vi "Logic.vi"(8 "error in (no error)":errorcluster, 11 "CIFTemplatePlugin in":refnum<class "CIFTemplatePlugin.lvclass">) -> (0 "error out":errorcluster, 3 "CIFTemplatePlugin out":refnum<class "CIFTemplatePlugin.lvclass">)   [LabVIEW 2021, in "CIFTemplatePlugin.lvclass"]
uses:
  CIFTemplatePlugin.lvclass
  D:/dev/CIF-LVCore/src/CIFCore/Class/CIFCorePlugin.lvclass
  CIFTemplatePlugin.lvclass/CIFTemplatePlugin.ctl
  Common/Typedef/Channels.ctl
  CIFCore/Class/CIFCorePlugin.lvclass/CIFCorePlugin.ctl
  Channels/CIFChannelMng/CIFChannelMng.lvclass/CIFChannelMng.ctl
  Channels/CIFChannels/CIFChannels.lvclass/CIFChannels.ctl
  Channels/CIFTag/Double/CIFTagDouble.lvclass/CIFTagDouble.ctl
  Channels/CIFTag/CIFTag/CIFTag.lvclass/CIFTag.ctl
  Channels/CIFTag/U64/CIFTagU64.lvclass/CIFTagU64.ctl
  CIFCore/Class/Accessors/Monitor/Write Double 1.vi
  CIFCore/Class/Accessors/Monitor/Write U64 1.vi
  CIFCore/Class/Accessors/Monitor/Write I64 1.vi
  CIFCore/Class/Accessors/Monitor/Write I64 2.vi
  Channels/CIFTag/CIFTag/Accessors/Read CIF Channel.vi
  Channels/CIFTag/CIFTag/SubVIs/Check Disconnect.vi
  Channels/CIFTag/Double/Core/Read Double_no_dd.vi/cbead010-ab61-49ec-ac6c-083511305d37.vi
  Channels/CIFTag/CIFTag/Accessors/Write CIF Channel.vi
  Channels/CIFChannels/Accessors/Read Channel State.vi
  Channels/CIFChannels/Accessors/Read Direction.vi
  Channels/CIFChannels/Accessors/Read Forced.vi
  Channels/CIFTag/U64/Core/Read U64_no_dd.vi/cbead010-ab61-49ec-ac6c-083511305d37.vi
  Channels/CIFTag/Double/Core/Write Double_no_dd.vi/e6e5dc56-0fe0-434b-816e-55c2e61471c2.vi
  Channels/CIFTag/U64/Core/Write U64_no_dd.vi/e6e5dc56-0fe0-434b-816e-55c2e61471c2.vi
  Channels/CIFChannels/Accessors/Write Channel State.vi
  Channels/CIFChannels/Accessors/Read Disconnect Behavior.vi
  Channels/CIFTag/Double/Core/Read Double_no_dd.vi/cbead010-ab61-49ec-ac6c-083511305d37.vi/c28b0ead-42ad-4072-80a2-aca7f2bd7ce3.vi
  Channels/CIFTag/Double/Core/Read Double_no_dd.vi/cbead010-ab61-49ec-ac6c-083511305d37.vi/219d0231-d98b-4193-b5cc-84f90e3c9091.vi
  <vilib>/CIFChannels/SubVIs/Get dll Path.vi
  Channels/CIFTag/U64/Core/Read U64_no_dd.vi/cbead010-ab61-49ec-ac6c-083511305d37.vi/c28b0ead-42ad-4072-80a2-aca7f2bd7ce3.vi
  Channels/CIFTag/U64/Core/Read U64_no_dd.vi/cbead010-ab61-49ec-ac6c-083511305d37.vi/219d0231-d98b-4193-b5cc-84f90e3c9091.vi
  Channels/CIFTag/Double/Core/Write Double_no_dd.vi/e6e5dc56-0fe0-434b-816e-55c2e61471c2.vi/4bc1c15b-36ab-481f-b8dd-c64075ce723a.vi
  Channels/CIFTag/Double/Core/Write Double_no_dd.vi/e6e5dc56-0fe0-434b-816e-55c2e61471c2.vi/d83cb72b-7713-41fc-a3d1-682de79cf574.vi
  Channels/CIFTag/U64/Core/Write U64_no_dd.vi/e6e5dc56-0fe0-434b-816e-55c2e61471c2.vi/4bc1c15b-36ab-481f-b8dd-c64075ce723a.vi
  Channels/CIFTag/U64/Core/Write U64_no_dd.vi/e6e5dc56-0fe0-434b-816e-55c2e61471c2.vi/d83cb72b-7713-41fc-a3d1-682de79cf574.vi
  Channels/CIFTag/CIFTag/CIFTag.lvclass
  D:/dev/CIF-LVCore/src/Channels/CIFChannels/CIFChannels.lvclass
  Channels/CIFChannelMng/CIFChannelMng.lvclass
  CIFCore/Class/CIFCorePlugin.lvclass
  Common/CIFTemplatePluginCommon.lvlib
  Channels/CIFTag/Double/CIFTagDouble.lvclass
  Channels/CIFTag/U64/CIFTagU64.lvclass
  D:/dev/CIF-LVCore/src/Channels/CIFTag/CIFTag/CIFTag.lvclass
  D:/dev/CIF-LVCore/src/Channels/CIFTag/Double/CIFTagDouble.lvclass
  D:/dev/CIF-LVCore/src/CIFTemplatePlugin/Class/CIFTemplatePlugin.lvclass
  D:/dev/CIF-LVCore/src/Channels/CIFTag/U64/CIFTagU64.lvclass
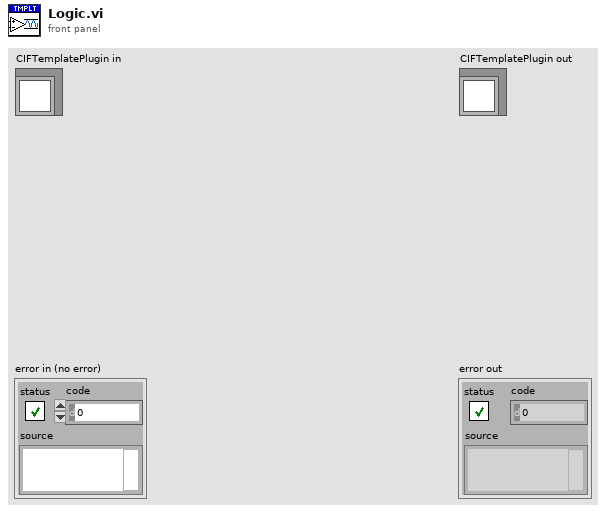
[diagram p1: front panel]
types:
  T1 = typedef "CIFTemplatePluginCommon.lvlib/Channels.ctl" = enum16{"doubleout", "doublein1", "doublein2", "uint_out", "uint_in"}
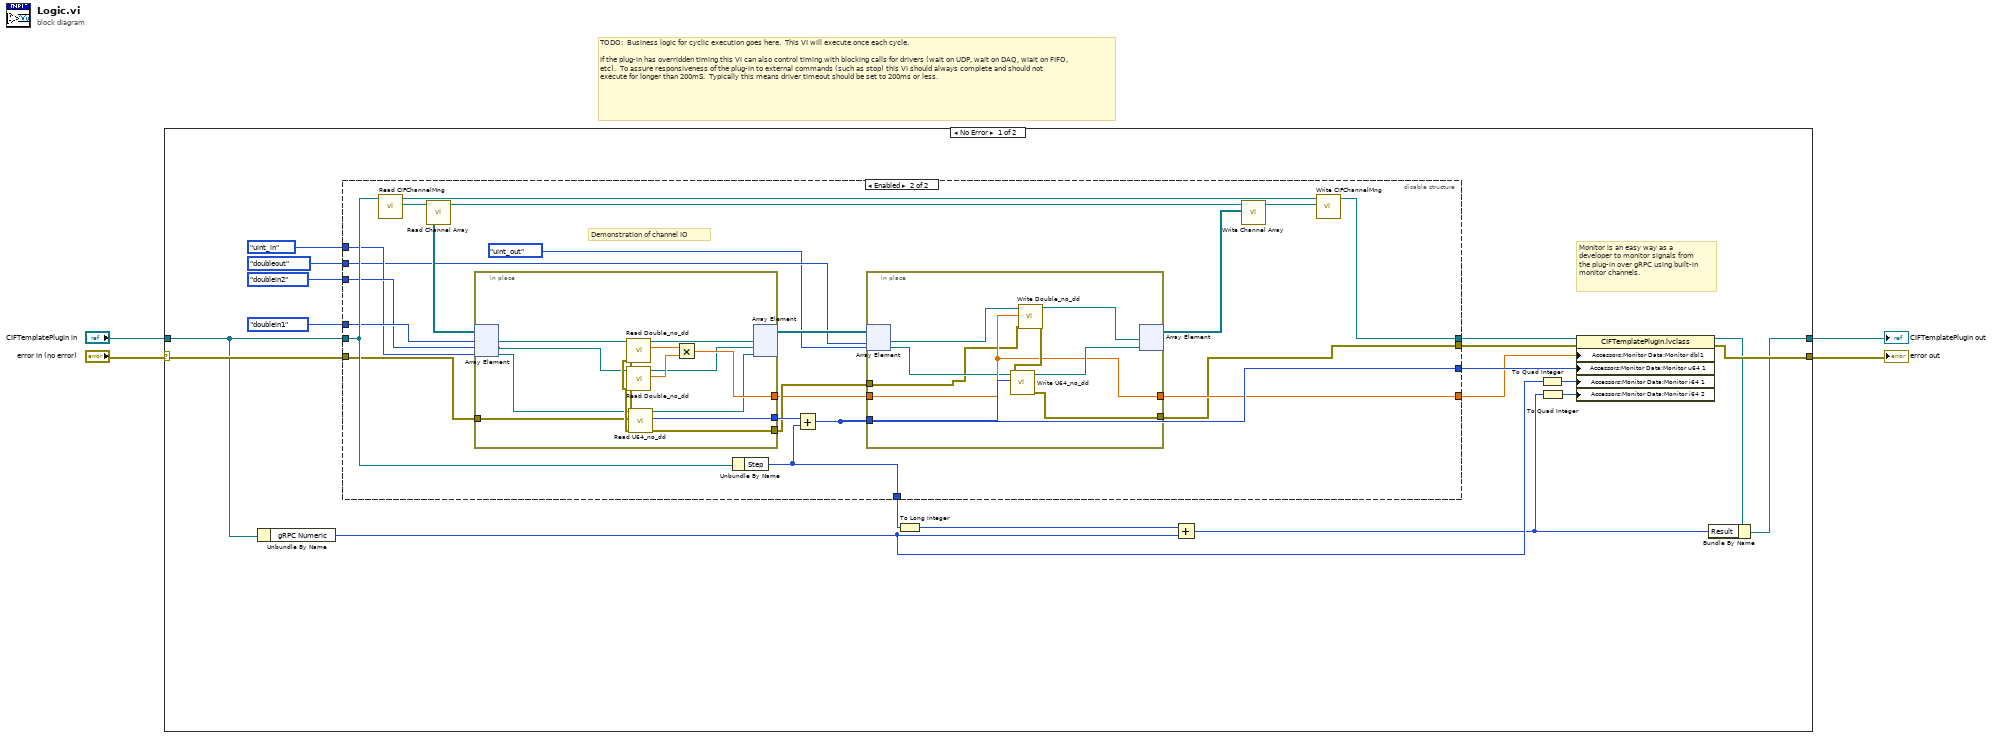
[diagram p0: block diagram]
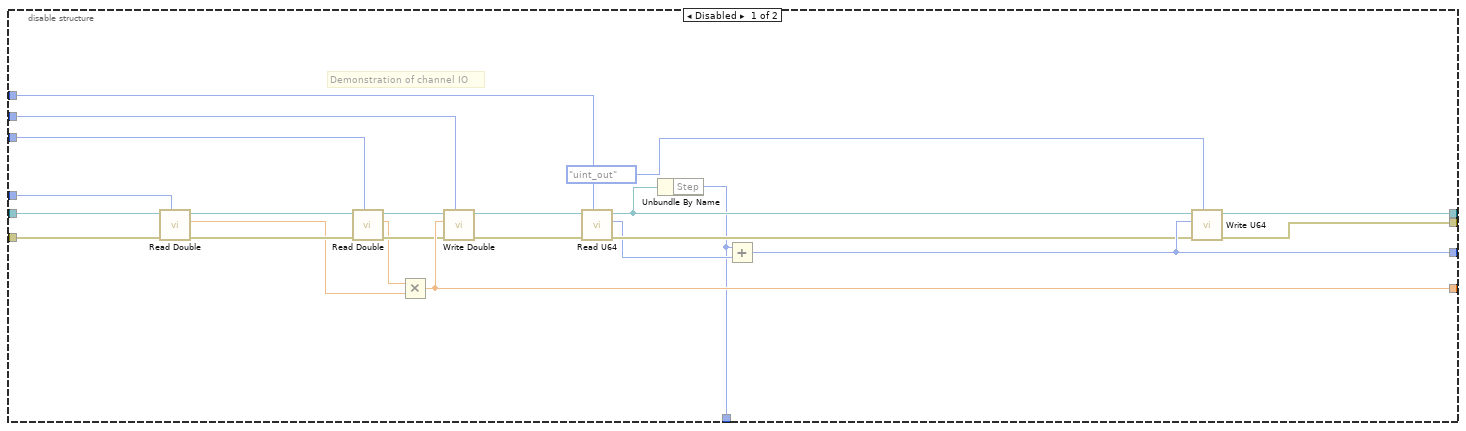
[diagram p2: hidden frame]
diagram:
  # "TODO:  Business logic for cyclic execution goes here.  This VI will execute once each cycle.  \n\nIf the plug-in has overridden timing this VI can also control timing with blocking calls for drivers (wait on UDP, wait on DAQ, wiait on FIFO, etc).  To assure responsiveness of the plug-in to external commands (such as stop) this VI should always complete and should not execute for longer than 200mS.  Typically this means driver timeout should be set to 200ms or less."
  n1 = case shown="No Error" "error in (no error)" {
    selector: "error in (no error)" -> [w23 w93]
    tunnel: [w22 w93] -> w3
    tunnel: [w5 w92] -> w1
    tunnel: "CIFTemplatePlugin in" -> [w7 w92]
    frame No Error {
      # "Monitor is an easy way as a developer to monitor signals from the plug-in over gRPC using built-in monitor channels."
      n2 = Unbundle By Name(w7) -> ("gRPC Numeric"=w11:i32)
      n3 = disable-structure shown="Enabled" {
        disable-tunnel: w23 -> [w46 w60]
        disable-tunnel: [w45 w48] -> w21
        disable-tunnel: [w44 w51] -> w20
        disable-tunnel: [w43 w53] -> w19
        disable-tunnel: [w42 w52] -> w18
        disable-tunnel: Channels."doublein1" ("Channels") -> [w33 w63]
        disable-tunnel: Channels."doublein2" ("Channels") -> [w32 w62]
        disable-tunnel: Channels."doubleout" ("Channels") -> [w31 w57]
        disable-tunnel: Channels."uint_in" ("Channels") -> [w30 w61]
        disable-tunnel: [w25 w68] -> w13
        disable-tunnel: w7 -> [w24 w65]
        frame Disabled {
          # "Demonstration of channel IO"
          n4 = call "Read Double.vi"("Channel Index"=w33, "error in (no error)"=w46, "CIFCorePlugin in"=w24) -> ("error out"=w39:errorcluster, "Data"=w36:dbl, "CIFCorePlugin out"=w41:refnum<class "CIFTemplatePlugin.lvclass">)  [unwired: 6 in]
          n5 = call "Read Double.vi"("Channel Index"=w32, "error in (no error)"=w39, "CIFCorePlugin in"=w41) -> ("error out"=w38:errorcluster, "Data"=w37:dbl, "CIFCorePlugin out"=w40:refnum<class "CIFTemplatePlugin.lvclass">)  [unwired: 6 in]
          n6 = Multiply(x=w37, y=w36) -> (x*y=w42:dbl)
          n7 = call "Write Double.vi"("Channel Index"=w31, "error in (no error)"=w38, "Data"=w42, "CIFCorePlugin in"=w40) -> ("error out"=w34:errorcluster, "CIFCorePlugin out"=w35:refnum<class "CIFTemplatePlugin.lvclass">)  [unwired: 6 in]
          n8 = call "Read U64.vi"("Channel Index"=w30, "error in (no error)"=w34, "CIFCorePlugin in"=w35) -> ("error out"=w29:errorcluster, "Data"=w27:u64, "CIFCorePlugin out"=w28:refnum<class "CIFTemplatePlugin.lvclass">)  [unwired: 6 in]
          n9 = Unbundle By Name(w28) -> ("Step"=w25:u64)
          n10 = Add(x=w25, y=w27) -> (x+y=w43:u64)
          n11 = call "Write U64.vi"("Channel Index"=Channels."uint_out" ("Channels"), "error in (no error)"=w29, "Data"=w43, "CIFCorePlugin in"=w28) -> ("error out"=w44:errorcluster, "CIFCorePlugin out"=w45:refnum<class "CIFTemplatePlugin.lvclass">)  [unwired: 6 in]
        }
        frame Enabled {
          # "Demonstration of channel IO"
          n12 = call "Read CIFChannelMng.vi"("CIFCorePlugin in"=w65) -> ("CIFChannelMng.lvclass"=w66:refnum<class "CIFChannelMng.lvclass">, "CIFCorePlugin out"=w47:refnum<class "CIFTemplatePlugin.lvclass">)  [unwired: 8 in, 1 out]
          n13 = call "Read Channel Array.vi"("CIFChannelMng in"=w66) -> ("Channel Array"=w64:refnum<class "CIFChannels.lvclass">[], "CIFChannelMng out"=w67:refnum<class "CIFChannelMng.lvclass">)  [unwired: 8 in, 1 out]
          n14 = in-place {
            in-place-border: [w90] -> w54
            in-place-border: [w85] -> w59
            in-place-border: w60 -> [w78]
            in-place-border: [w82] -> w55
            n15 = in-place-array #1(w64, w63, w62, w61) -> (w81:refnum<class "CIFChannels.lvclass">, w80:refnum<class "CIFChannels.lvclass">, w79:refnum<class "CIFChannels.lvclass">)
            n16 = call "Read Double_no_dd.vi"("error in (no error)"=w78, "CIFTag in"=w81) -> ("error out"=w84:errorcluster, "Data"=w91:dbl, "CIFTag out"=w88:refnum<class "CIFTagDouble.lvclass">)  [unwired: 6 in, 1 out]
            n17 = call "Read Double_no_dd.vi"("error in (no error)"=w84, "CIFTag in"=w80) -> ("error out"=w83:errorcluster, "Data"=w89:dbl, "CIFTag out"=w87:refnum<class "CIFTagDouble.lvclass">)  [unwired: 6 in, 1 out]
            n18 = call "Read U64_no_dd.vi"("error in (no error)"=w83, "CIFTag in"=w79) -> ("error out"=w82:errorcluster, "Data"=w85:u64, "CIFTag out"=w86:refnum<class "CIFTagU64.lvclass">)  [unwired: 6 in, 1 out]
            n19 = Multiply(x=w91, y=w89) -> (x*y=w90:dbl)
            n20 = in-place-array #1(w88, w87, w86) -> (w58:refnum<class "CIFChannels.lvclass">[])  [unwired: 3 out]
          }
          n21 = Unbundle By Name(w65) -> ("Step"=w68:u64)
          n22 = Add(x=w59, y=w68) -> (x+y=w53:u64)
          n23 = in-place {
            in-place-border: [w72] -> w52
            in-place-border: w55 -> [w69]
            in-place-border: w54 -> [w72]
            in-place-border: w53 -> [w76]
            in-place-border: [w73] -> w51
            n24 = in-place-array #2(w58, w57, Channels."uint_out" ("Channels")) -> (w71:refnum<class "CIFChannels.lvclass">, w70:refnum<class "CIFChannels.lvclass">)
            n25 = call "Write Double_no_dd.vi"("error in (no error)"=w69, "Data"=w72, "CIFTag in"=w71) -> ("error out"=w77:errorcluster, "CIFTag out"=w75:refnum<class "CIFTagDouble.lvclass">)  [unwired: 6 in, 1 out]
            n26 = call "Write U64_no_dd.vi"("error in (no error)"=w77, "Data"=w76, "CIFTag in"=w70) -> ("error out"=w73:errorcluster, "CIFTag out"=w74:refnum<class "CIFTagU64.lvclass">)  [unwired: 6 in, 1 out]
            n27 = in-place-array #2(w75, w74) -> (w50:refnum<class "CIFChannels.lvclass">[])  [unwired: 2 out]
          }
          n28 = call "Write Channel Array.vi"("Channel Array"=w50, "CIFChannelMng in"=w67) -> ("CIFChannelMng out"=w49:refnum<class "CIFChannelMng.lvclass">)  [unwired: 8 in, 1 out]
          n29 = call "Write CIFChannelMng.vi"("CIFChannelMng.lvclass"=w49, "CIFCorePlugin in"=w47) -> ("CIFCorePlugin out"=w48:refnum<class "CIFTemplatePlugin.lvclass">)  [unwired: 8 in, 1 out]
        }
      }
      n30 = To Long Integer(number=w13) -> (32bit integer=w12:i32)
      n31 = Add(x=w12, y=w11) -> (x+y=w10:i32)
      n32 = To Quad Integer(1:w11) -> (0:w9:i64)
      n33 = To Quad Integer(1:w10) -> (0:w8:i64)
      n34 = property class="CIFTemplatePlugin.lvclass"(reference=w21, error in=w20, "Accessors:Monitor Data:Monitor dbl1"=w18, "Accessors:Monitor Data:Monitor u64 1"=w19, "Accessors:Monitor Data:Monitor i64 1"=w9, "Accessors:Monitor Data:Monitor i64 2"=w8) -> (reference out=w6:refnum<class "CIFTemplatePlugin.lvclass">, error out=w22:errorcluster)
      n35 = Bundle By Name(cluster=w6, "Result"=w10) -> (w5:refnum<class "CIFTemplatePlugin.lvclass">)
    }
    frame Error {
    }
  }
  "error out" <- w3
  "CIFTemplatePlugin out" <- w1
